vi "create.s3path.vi"(10 "path":string) -> (3 "Timestamp Manifest":refnum<class "s3path.lvclass">)   [LabVIEW 2020, in "nominal types.lvlib" / "timestampManifest.lvlib"]
uses:
  timestampManifest.lvlib
  s3path/s3path.lvclass
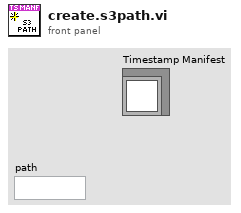
[diagram p1: front panel]
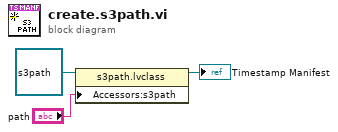
[diagram p0: block diagram]
diagram:
  n1 = property class="s3path.lvclass"(reference=refnum<class "s3path.lvclass"> refnum ("nominal types.lvlib:timestampManifest.lvlib:s3path.lvclass"), "Accessors:s3path"="path") -> (reference out=→"Timestamp Manifest":refnum<class "s3path.lvclass">)  [unwired: 1 in, 1 out]
